vi "p6.vi"() -> ()   [LabVIEW 2015]
panel:
  out "shift reg 1":i32
  out "shift reg 2":i32
  out "i":i32
  out "inside loop":i32
  out "appended array 2":string[](array[string])
  out "size(s)":i32
  out "with name cluster":cluster{"Numeric 1":dbl, "Numeric 2":dbl}
  out "without name cluster":cluster{dbl, dbl}
  in  "Cluster":cluster{"Numeric 1":dbl, "Numeric 2":dbl}
  out "unsigned 16bit integer":u16
  out "unsigned 8bit integer":u8
  out "In Range?":bool
  out "coerced(x)":dbl
  out "number":u32
  in  "Array 2":bool[](array[boolean])
  out "8 bit integer":u8
  out "64bit integer":i64
  out "appended array":i32[](array[numeric])
  out "Boolean":bool
  in  "Array":bool[](array[boolean])
  # "EXAMPLE 5"
  # "EXAMPLE 2"
  # "EXAMPLE 4"
  # "EXAMPLE 6"
  # "EXAMPLE 3"
  # "EXAMPLE 1"
  # "EXAMPLE 7"
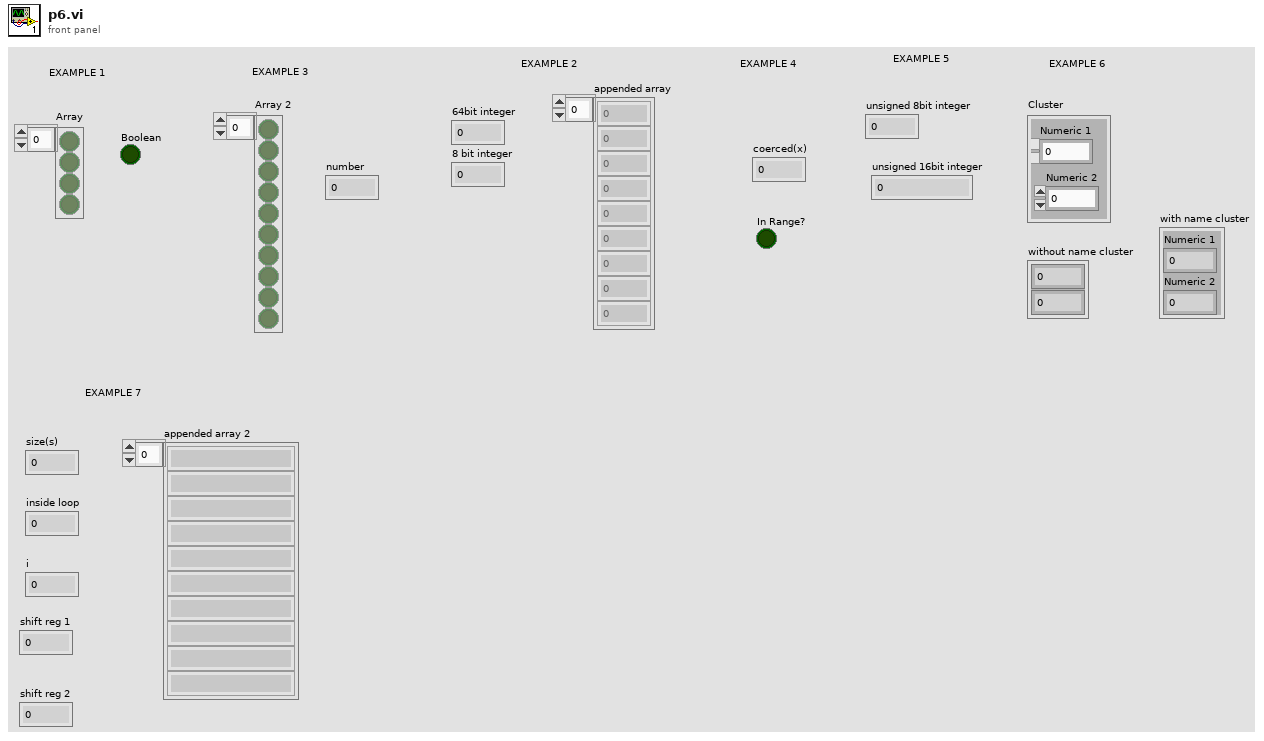
[diagram p1: front panel]
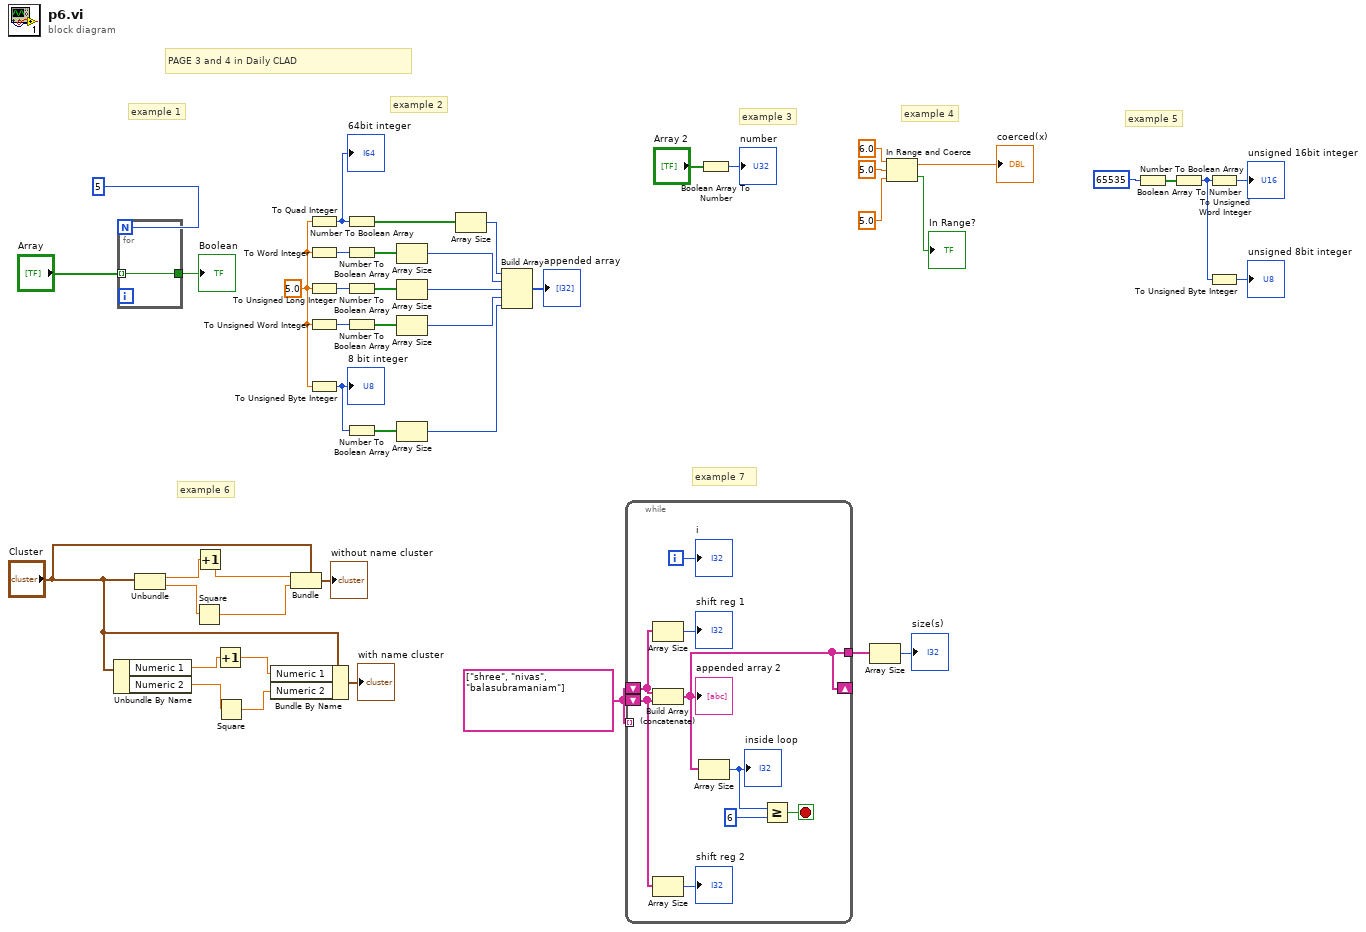
[diagram p0: block diagram]
diagram:
  w3 = string[] ["shree", "nivas", "balasubramaniam"] ("Array 3")
  w43 = 5.0
  # "example 7"
  # "PAGE 3 and 4 in Daily CLAD"
  # "example 6"
  # "example 5"
  # "example 4"
  # "example 3"
  # "example 2"
  # "example 1"
  n1 = Unbundle By Name("Cluster") -> ("Numeric 1"=w9:dbl, "Numeric 2"=w8:dbl)
  n2 = for {
    N: 5 -> [_]
    tunnel: "Array" -> [w47] mode=indexing
    tunnel: [w47] -> w44
  }
  "Boolean" <- w44
  n3 = Unbundle("Cluster") -> ("Numeric 1"=w12:dbl, "Numeric 2"=w11:dbl)
  n4 = Square(x=w11) -> (x^2=w14:dbl)
  n5 = Increment(x=w12) -> (x+1=w13:dbl)
  n6 = Increment(x=w9) -> (x+1=w6:dbl)
  n7 = Square(x=w8) -> (x^2=w5:dbl)
  n8 = Bundle By Name(cluster="Cluster", "Numeric 1"=w6, "Numeric 2"=w5) -> (→"with name cluster":cluster{"Numeric 1":dbl, "Numeric 2":dbl})
  n9 = Bundle(cluster="Cluster", "Numeric 1"=w13, "Numeric 2"=w14) -> (→"without name cluster":cluster{"Numeric 1":dbl, "Numeric 2":dbl})
  n10 = To Quad Integer(1:w43) -> (0:w39:i64)
  "64bit integer" <- w39
  n11 = To Word Integer(number=w43) -> (16bit integer=w40:i16)
  n12 = To Unsigned Long Integer(number=w43) -> (unsigned 32bit integer=w41:u32)
  n13 = To Unsigned Word Integer(number=w43) -> (unsigned 16bit integer=w42:u16)
  n14 = To Unsigned Byte Integer(number=w43) -> (unsigned 8bit integer=w27:u8)
  "8 bit integer" <- w27
  n15 = Number To Boolean Array(number=w39) -> (Boolean array=w38:bool[])
  n16 = Number To Boolean Array(number=w40) -> (Boolean array=w37:bool[])
  n17 = Number To Boolean Array(number=w41) -> (Boolean array=w36:bool[])
  n18 = Number To Boolean Array(number=w42) -> (Boolean array=w35:bool[])
  n19 = Number To Boolean Array(number=w27) -> (Boolean array=w34:bool[])
  n20 = Array Size(array=w37) -> (size(s)=w32:i32)
  n21 = Array Size(array=w36) -> (size(s)=w31:i32)
  n22 = Array Size(array=w35) -> (size(s)=w30:i32)
  n23 = Array Size(array=w34) -> (size(s)=w29:i32)
  n24 = Array Size(array=w38) -> (size(s)=w33:i32)
  n25 = Build Array(w33, w32, w31, w30, w29) -> (→"appended array":i32[])
  n26 = while {
    shift-right: [w53] -> _
    shift-left: w3 -> [w48]
    shift-left: w3 -> [w51]
    tunnel: w3 -> [_] mode=indexing
    tunnel: [w53] -> w2
    i -> [w52]
    stop <- w54 stop-if-true
    n27 = Array Size(array=w48) -> (size(s)=→"shift reg 1":i32)
    n28 = Build Array (concatenate)(w48, w51) -> (w53:string[])
    "appended array 2" <- w53
    n29 = Array Size(array=w51) -> (size(s)=→"shift reg 2":i32)
    n30 = Array Size(array=w53) -> (size(s)=w56:i32)
    "inside loop" <- w56
    n31 = Greater Or Equal?(x=w56, y=6) -> (x >= y?=w54:bool)
    "i" <- w52
  }
  n32 = Boolean Array To Number(Boolean array="Array 2") -> (number=→"number":u32)
  n33 = Array Size(array=w2) -> (size(s)=→"size(s)":i32)
  n34 = In Range and Coerce(upper limit=6.0, x=5.0, lower limit=5.0) -> (coerced(x)=→"coerced(x)":dbl, In Range?=→"In Range?":bool)
  n35 = Number To Boolean Array(number=u32 65535) -> (Boolean array=w19:bool[])
  n36 = Boolean Array To Number(Boolean array=w19) -> (number=w17:u32)
  n37 = To Unsigned Word Integer(number=w17) -> (unsigned 16bit integer=→"unsigned 16bit integer":u16)
  n38 = To Unsigned Byte Integer(number=w17) -> (unsigned 8bit integer=→"unsigned 8bit integer":u8)
